vi "Tray_main_glbRef.vi"() -> ()   [LabVIEW 2015]
panel:
  in  "Main_SeverReply":refnum<vi>
  out "Main_MsgRef":refnum<vi>[](array[refnum])
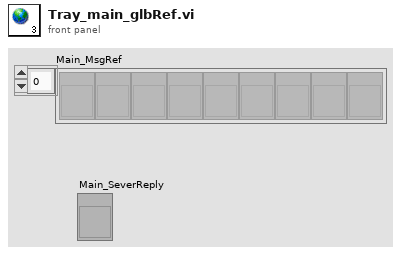
[diagram p1: front panel]
diagram:
